vi "Difference In Time.vi"(11 "x-y":dbl) -> ()   [LabVIEW 2023]
panel:
  out "Hours":i64
  out "Days":i64
  out "Minuites":i64
  out "Seconds":i64
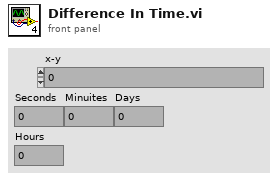
[diagram p1: front panel]
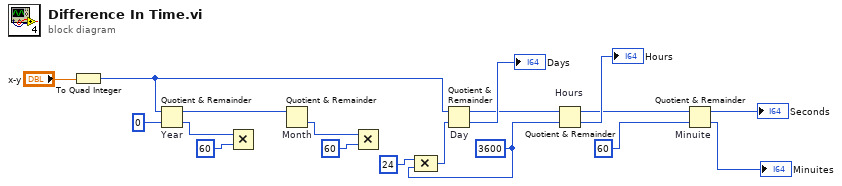
[diagram p0: block diagram]
diagram:
  w1 = i64 3600 ("y")
  n1 = To Quad Integer(1:"x-y") -> (0:w9:i64)
  n2 = Quotient & Remainder "Year"(x=w9, y=i64 0) -> (x-y*floor(x/y)=w4:i64, floor(x/y)=w15:i64)
  n3 = Multiply(x=w15, y=i64 60) -> ()  [unwired: 1 out]
  n4 = Quotient & Remainder "Month"(x=w4) -> (floor(x/y)=w14:i64)  [unwired: 1 in, 1 out]
  n5 = Multiply(x=w14, y=i64 60) -> ()  [unwired: 1 out]
  n6 = Compound Arithmetic op=MULTIPLY(i64 24 ("y"), w1) -> (w3:i64)
  n7 = Quotient & Remainder "Day"(x=w9, y=w3) -> (x-y*floor(x/y)=w7:i64, floor(x/y)=→"Days":i64)
  n8 = Quotient & Remainder "Hours"(x=w7, y=w1) -> (x-y*floor(x/y)=w5:i64, floor(x/y)=→"Hours":i64)
  n9 = Quotient & Remainder "Minuite"(x=w5, y=i64 60) -> (x-y*floor(x/y)=→"Seconds":i64, floor(x/y)=→"Minuites":i64)
